vi "To MotorPWM.vi"(2 "error in (no error)":errorcluster, 3 "Speed":dbl, 4 "Car.lvclass":refnum<class "Car.lvclass">) -> (0 "error out":errorcluster, 1 "MotorPWM":dbl)   [LabVIEW 2015, in "Car.lvclass"]
uses:
  Car.lvclass
  Car.lvclass/Car.ctl
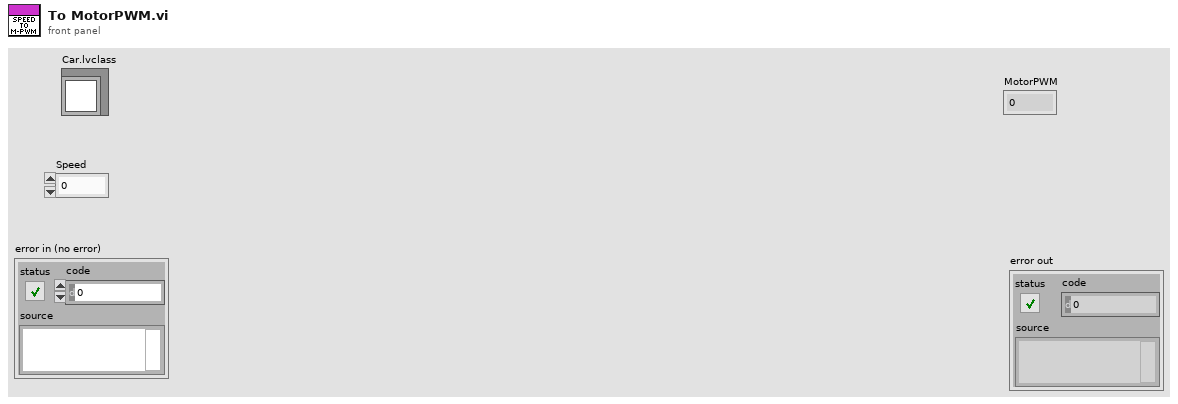
[diagram p1: front panel]
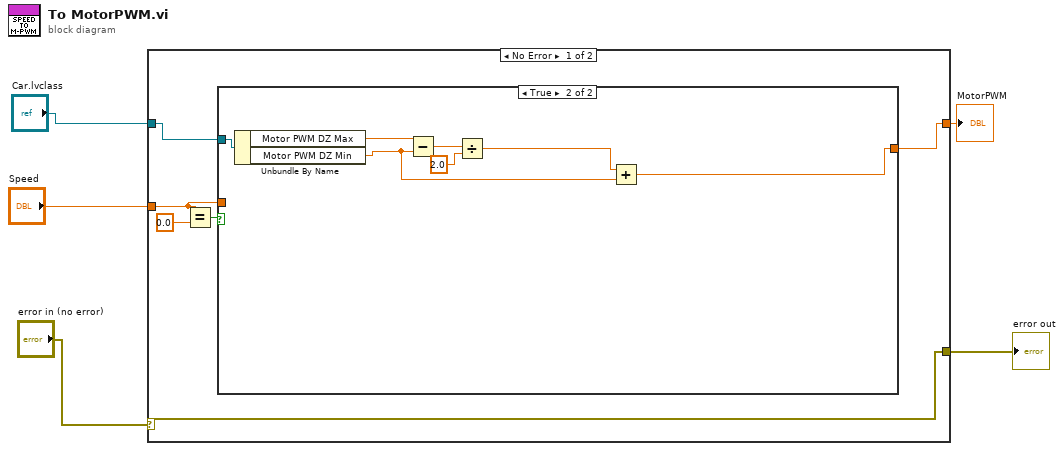
[diagram p0: block diagram]
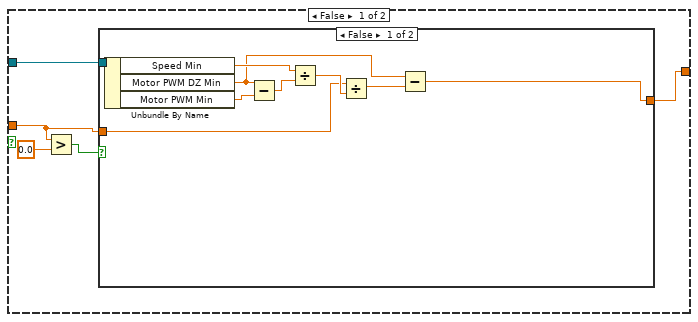
[diagram p2: hidden frame]
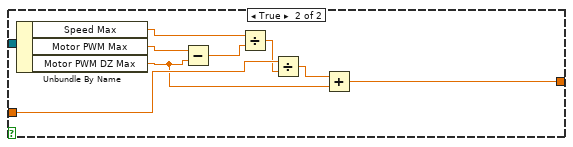
[diagram p3: hidden frame]
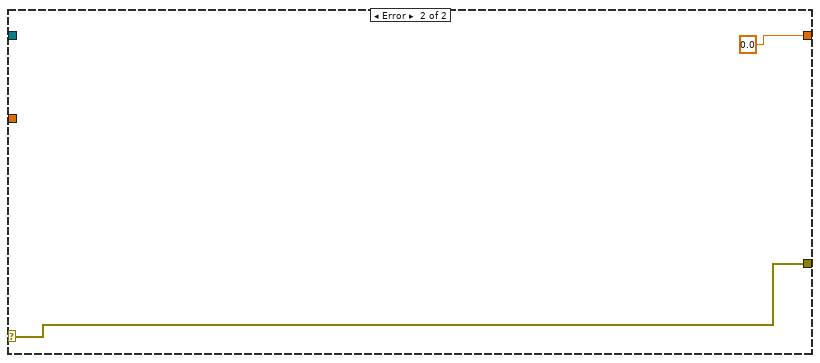
[diagram p4: hidden frame]
diagram:
  n1 = case shown="No Error" "error in (no error)" {
    selector: "error in (no error)" -> [w11 w43]
    tunnel: [w11 w43] -> w4
    tunnel: [w6 0.0] -> w3
    tunnel: "Car.lvclass" -> [w7 _]
    tunnel: "Speed" -> [w8 _]
    frame No Error {
      n2 = Equal?(x=w8, y=0.0) -> (x = y?=w9:bool)
      n3 = case shown="True" w9 {
        tunnel: w8 -> [w13 _]
        tunnel: w7 -> [w14 w41]
        tunnel: [w12 w35] -> w6
        frame False {
          n4 = Greater?(x=w13, y=0.0) -> (0:w15:bool)
          n5 = case shown="False" w15 {
            tunnel: w14 -> [w25 w34]
            tunnel: w13 -> [w20 w30]
            tunnel: [w17 w26] -> w12
            frame False {
              n6 = Unbundle By Name(w25) -> ("Speed Min"=w23:dbl, "Motor PWM DZ Min"=w18:dbl, "Motor PWM Min"=w24:dbl)
              n7 = Subtract(x=w18, y=w24) -> (x-y=w22:dbl)
              n8 = Divide(x=w23, y=w22) -> (x/y=w21:dbl)
              n9 = Divide(x=w20, y=w21) -> (x/y=w19:dbl)
              n10 = Subtract(x=w18, y=w19) -> (x-y=w17:dbl)
            }
            frame True {
              n11 = Unbundle By Name(w34) -> ("Speed Max"=w32:dbl, "Motor PWM Max"=w33:dbl, "Motor PWM DZ Max"=w27:dbl)
              n12 = Subtract(x=w33, y=w27) -> (x-y=w31:dbl)
              n13 = Divide(x=w32, y=w31) -> (x/y=w29:dbl)
              n14 = Divide(x=w30, y=w29) -> (x/y=w28:dbl)
              n15 = Add(x=w28, y=w27) -> (x+y=w26:dbl)
            }
          }
        }
        frame True {
          n16 = Unbundle By Name(w41) -> ("Motor PWM DZ Max"=w40:dbl, "Motor PWM DZ Min"=w37:dbl)
          n17 = Subtract(x=w40, y=w37) -> (x-y=w38:dbl)
          n18 = Divide(x=w38, y=2.0) -> (x/y=w36:dbl)
          n19 = Add(x=w36, y=w37) -> (x+y=w35:dbl)
        }
      }
    }
    frame Error {
    }
  }
  "error out" <- w4
  "MotorPWM" <- w3
